vi "Replace Chan Grp.vi"(8 "error in (no error)":errorcluster, 9 "ChanGroupPos":i32, 10 "ChanGrp to Add":refnum<class "ChanGrp.lvclass">, 11 "TimingGrp in":refnum<class "TimingGrp.lvclass">) -> (0 "error out":errorcluster, 3 "TimingGrp out":refnum<class "TimingGrp.lvclass">)   [LabVIEW 2018, in "Configuration Grandmaster.lvlib" / "TimingGrp.lvclass"]
uses:
  TimingGrp.lvclass
  Class Chan Group/ChanGrp.lvclass
  TimingGrp.lvclass/TimingGrp.ctl
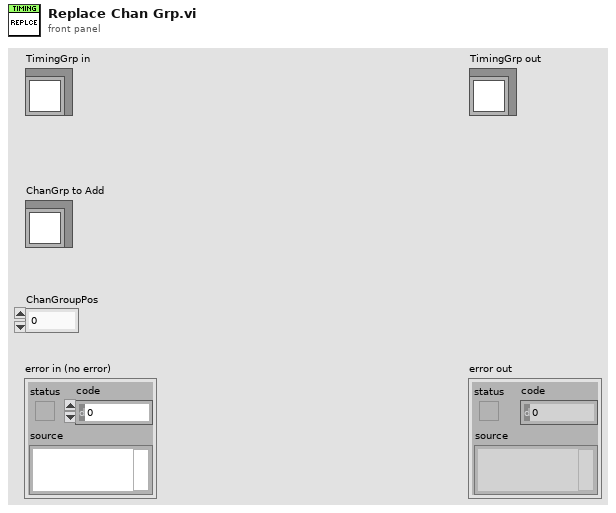
[diagram p1: front panel]
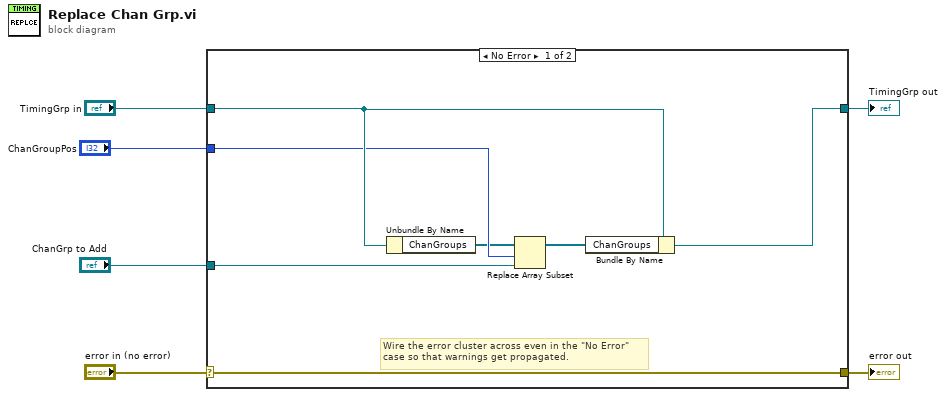
[diagram p0: block diagram]
diagram:
  n1 = case shown="No Error" "error in (no error)" {
    selector: "error in (no error)" -> [w13 w15]
    tunnel: [w13 w15] -> w5
    tunnel: [w11 w14] -> w3
    tunnel: "TimingGrp in" -> [w10 w14]
    tunnel: "ChanGrp to Add" -> [w12 _]
    tunnel: "ChanGroupPos" -> [w9 _]
    frame No Error {
      # "Wire the error cluster across even in the \"No Error\"\ncase so that warnings get propagated."
      n2 = Unbundle By Name(w10) -> ("ChanGroups"=w8:refnum<class "ChanGrp.lvclass">[])
      n3 = Replace Array Subset(array=w8, new element=w12, index=w9) -> (w7:refnum<class "ChanGrp.lvclass">[])
      n4 = Bundle By Name(cluster=w10, "ChanGroups"=w7) -> (w11:refnum<class "TimingGrp.lvclass">)
    }
    frame Error {
    }
  }
  "error out" <- w5
  "TimingGrp out" <- w3
